vi "WrapperWiresmith.vi"() -> ()   [LabVIEW 2019]
uses:
  b66d7838-5639-461a-bd18-8123a88c45dd.vi
  <vilib>/Wiresmith Technology/G CLI/CLI Class/CLI.lvclass
panel:
  out "error out":errorcluster
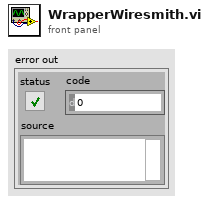
[diagram p1: front panel]
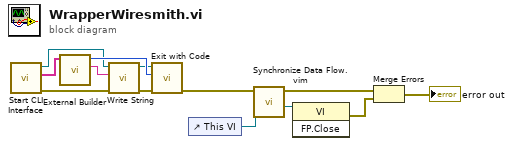
[diagram p0: block diagram]
diagram:
  n1 = call <vilib>:"Start CLI Interface.vi"() -> ("error out"=w10:errorcluster, "Custom Parameters"=w13:string[], "CLI out"=w7:refnum<class "CLI.lvclass">)  [unwired: 8 in, 1 out]
  n2 = call "External Builder.vi"("Arguments"=w13) -> ("Log String"=w11:string, "Return Code"=w12:i32)  [unwired: 9 in]
  n3 = call <vilib>:"Write String.vi"("error in (no error)"=w10, "Text to Write"=w11, "CLI in"=w7) -> ("error out"=w9:errorcluster, "CLI out"=w8:refnum<class "CLI.lvclass">)  [unwired: 7 in]
  n4 = call <vilib>:"Exit with Code.vi"("error in (no error)"=w9, "Exit Code (0)"=w12, "CLI in"=w8) -> ("error out"=w2:errorcluster)  [unwired: 8 in]
  n5 = control-ref of="This VI"() -> (w4:refnum<vi>)
  n6 = call "Synchronize Data Flow.vim"("input 3"=w4, "input 1"=w2) -> ("output 3"=w3:refnum<vi>, "output 1"=w1:errorcluster)  [unwired: 2 in, 2 out]
  n7 = invoke class="VI" method="FP.Close"(reference=w3) -> (error out=w6:errorcluster)  [unwired: 2 in, 2 out]
  n8 = Merge Errors(w1, w6) -> (→"error out":errorcluster)
